vi "WriteCtrlAttrListGen.vi"(4 "Error in":errorcluster, 6 "Attribut":string="DisAtStartup", 7 "Controls":refnum<vi>[](array[refnum])) -> (0 "Error out":errorcluster, 3 "Controls Out":refnum<vi>[](array[refnum]))   [LabVIEW 2010]
doc: "Ce VI ouvre le fichier de sauvegarde des modèles et lit les positions du modèle spécifié."
uses:
  <vilib>/Utility/config.llb/Write Key (String).vi
  <vilib>/Utility/config.llb/NI_LVConfig.lvlib
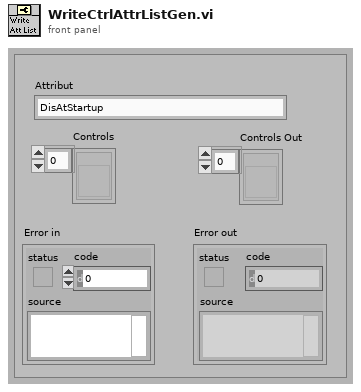
[diagram p1: front panel]
types:
  T1 = typedef "NI_LVConfig.lvlib/Config Data RefNum.ctl" = refnum<k1>
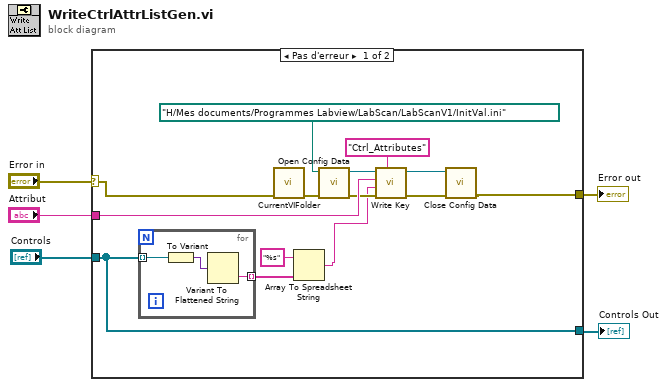
[diagram p0: block diagram]
diagram:
  n1 = case shown="Pas d'erreur" "Error in" {
    selector: "Error in" -> [w11 w24]
    tunnel: [w7 w24] -> w5
    tunnel: [w6 w23] -> w3
    tunnel: "Controls" -> [w6 w23]
    tunnel: "Attribut" -> [w14 _]
    frame No Error {
      n2 = for {
        tunnel: w6 -> [w21] mode=indexing
        tunnel: [w20] -> w10 mode=indexing
        n3 = To Variant(anything=w21) -> (Variant=w22:variant)
        n4 = Variant To Flattened String(Variant=w22) -> (data string=w20:string)  [unwired: 1 out]
      }
      n5 = call <userlib>:"CurrentVIFolder.vi"("error in (no error)"=w11) -> ("error out"=w19:errorcluster)  [unwired: 8 in, 2 out]
      n6 = Array To Spreadsheet String(array=w10, 3:"%s" ("chaîne de format")) -> (spreadsheet string=w8:string)  [unwired: 1 in]
      n7 = call <vilib>:"Open Config Data.vi"("error in (no error)"=w19, "configuration file path"=path "H:/Mes documents/Programmes Labview/LabScan/LabScanV1/InitVal.ini" ("chemin du VI")) -> ("error out"=w13:errorcluster, "refnum"=w17:T1)  [unwired: 7 in, 1 out]
      n8 = call-poly <vilib>:"Write Key.vi"("section"="Ctrl_Attributes", "error in (no error)"=w13, "value"=w8, "key"=w14, "refnum"=w17) -> ("error out"=w12:errorcluster, "refnum out"=w15:T1)  [unwired: 4 in, 1 out]
      n9 = call <vilib>:"Close Config Data.vi"("error in (no error)"=w12, "refnum"=w15) -> ("error out"=w7:errorcluster)  [unwired: 8 in, 1 out]
    }
    frame Error {
    }
  }
  "Error out" <- w5
  "Controls Out" <- w3
